vi "Fetch Measurement (Effective Temperature).vi"(8 "error in (no error)":errorcluster, 10 "Measurement Type (0: Corrected)":u16(ring) items=["Corrected", "Uncorrected"], 11 "VISA resource name":refnum<visa-resource-name>) -> (0 "error out":errorcluster, 2 "Effective Temperature Results (K)":dbl[](array[numeric]), 3 "VISA resource name out":refnum<visa-resource-name>)   [LabVIEW 2014, in "Agilent ESA PSA Series.lvlib"]
doc: "Returns the results of the last measurement (Effective Temperature) and does not initiate data acquisition.\n\n<B>Note:</B>\n\nThis VI is only valid for the Noise Figure functionality of the Noise Figure personality."
uses:
  Agilent ESA PSA Series.lvlib
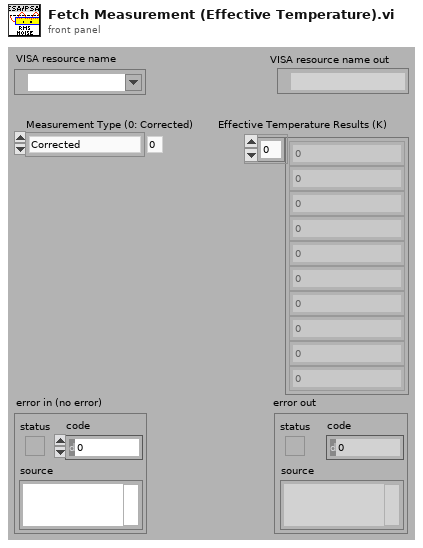
[diagram p1: front panel]
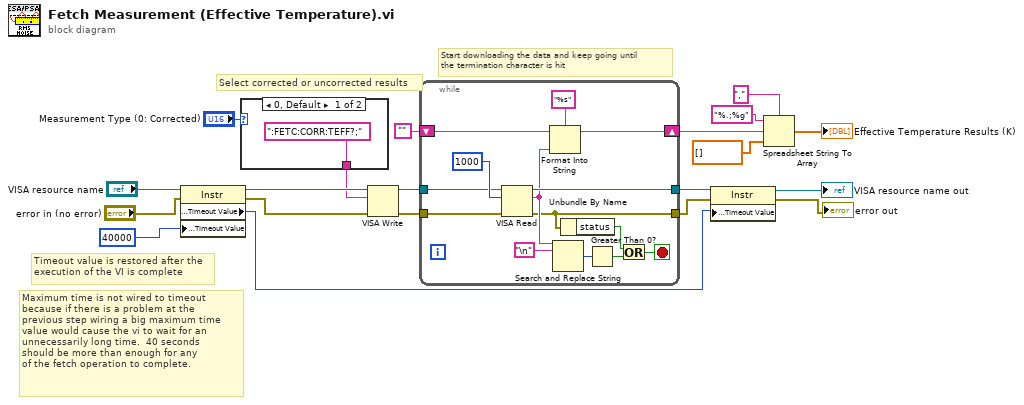
[diagram p0: block diagram]
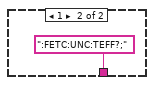
[diagram p2: hidden frame]
diagram:
  # "Select corrected or uncorrected results"
  # "Maximum time is not wired to timeout\nbecause if there is a problem at the\nprevious step wiring a big maximum time\nvalue would cause the vi to wait for an\nunnecessarily long time.  40 seconds\nshould be more than enough for any\nof the fetch operation to complete."
  # "Timeout value is restored after the\nexecution of the VI is complete"
  # "Start downloading the data and keep going until\nthe termination character is hit"
  n1 = property on="Property Node" class="Instr"(reference="VISA resource name", error in="error in (no error)", "General Settings:Timeout Value"=u32 40000) -> (reference out=w17:refnum<visa-resource-name>, error out=w18:errorcluster, "General Settings:Timeout Value"=w14:u32)
  n2 = case shown="0, Default" "Measurement Type (0: Corrected)" {
    tunnel: [":FETC:CORR:TEFF?;" ("string (\"\")") ":FETC:UNC:TEFF?;" ("string (\"\")")] -> w2
    frame 0, Default {
    }
    frame 1 {
    }
  }
  n3 = VISA Write(VISA resource name=w17, write buffer=w2, error in (no error)=w18) -> (VISA resource name out=w8:refnum<visa-resource-name>, error out=w7:errorcluster)  [unwired: 1 out]
  n4 = while {
    tunnel: [w35] -> w16
    tunnel: [w25] -> w15
    tunnel: w8 -> [w34]
    tunnel: w7 -> [w33]
    shift-right: [w29] -> w5
    shift-left: "" -> [w28]
    stop <- w24 stop-if-true
    n5 = VISA Read(VISA resource name=w34, byte count=u32 1000, error in (no error)=w33) -> (VISA resource name out=w35:refnum<visa-resource-name>, read buffer=w30:string, error out=w25:errorcluster)  [unwired: 1 out]
    n6 = Format Into String(format string="%s", initial string=w28, w30) -> (resulting string=w29:string)  [unwired: 1 in, 1 out]
    n7 = Search and Replace String(input string=w30, search string="\n") -> (number of replacements=w31:i32)  [unwired: 6 in, 3 out]
    n8 = Unbundle By Name(w25) -> ("status"=w26:bool)
    n9 = Greater Than 0?(x=w31) -> (x > 0?=w23:bool)
    n10 = Or(x=w26, y=w23) -> (x .or. y?=w24:bool)
  }
  n11 = property on="Property Node" class="Instr"(reference=w16, error in=w15, "General Settings:Timeout Value"=w14) -> (reference out=→"VISA resource name out":refnum<visa-resource-name>, error out=→"error out":errorcluster)
  n12 = Spreadsheet String To Array(delimiter (Tab)=",", format string="%.;%g", spreadsheet string=w5, array type (2D Dbl)=dbl[] []) -> (array=→"Effective Temperature Results (K)":dbl[])
